vi "Error Converter (ErrCode or Status).vi"(8 "error in (no error)":errorcluster, 11 "error code":i32) -> (0 "error out":errorcluster)   [LabVIEW 2023, in "uhd.lvlib"]
uses:
  <userlib>/uhd/uhd.lvlib
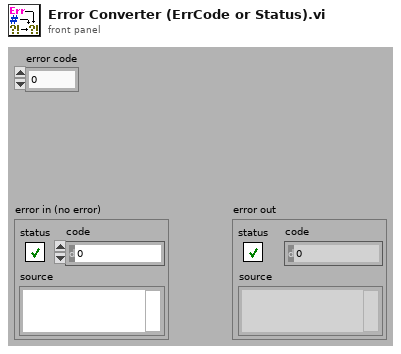
[diagram p1: front panel]
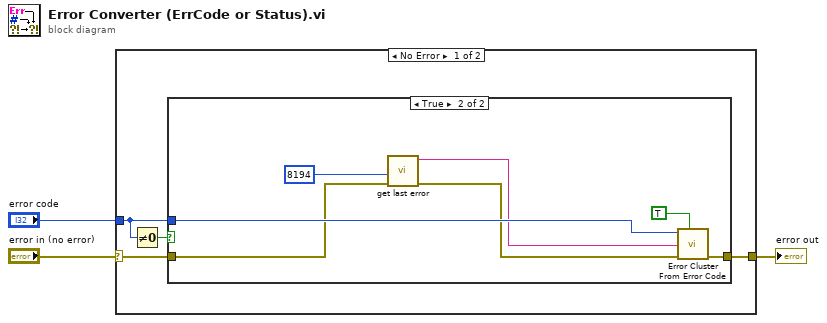
[diagram p0: block diagram]
diagram:
  n1 = case shown="No Error" "error in (no error)" {
    selector: "error in (no error)" -> [w6 w16]
    tunnel: [w4 w16] -> w2
    tunnel: "error code" -> [w5 _]
    frame No Error {
      n2 = Not Equal To 0?(x=w5) -> (x != 0?=w7:bool)
      n3 = case shown="True" w7 {
        tunnel: w6 -> [w8 w12]
        tunnel: w5 -> [_ w14]
        tunnel: [w8 w15] -> w4
        frame False {
        }
        frame True {
          n4 = call <userlib>:"get last error.vi"("error in (no error)"=w12, "strbuffer_len"=u64 8194) -> ("error out"=w9:errorcluster, "error_out out"=w10:string)  [unwired: 7 in, 1 out]
          n5 = call <vilib>:"Error Cluster From Error Code.vi"("show call chain? (False)"=TRUE, "error in (no error)"=w9, "error message (\"\")"=w10, "error code (0)"=w14) -> ("error out"=w15:errorcluster)  [unwired: 5 in]
        }
      }
    }
    frame Error {
    }
  }
  "error out" <- w2
